vi "pf Init Usb.vi"(8 "error in (no error)":errorcluster, 11 "pDllName":string) -> (0 "error out":errorcluster, 2 "function return":i32, 3 "pDllName out":string)   [LabVIEW 2025, in "Photonfocus_Toolkit.lvlib"]
doc: "PFCONFIG_API int pfInitUsb(char* pDllName);"
uses:
  Photonfocus_Toolkit.lvlib
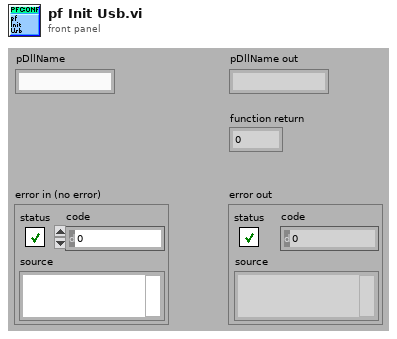
[diagram p1: front panel]
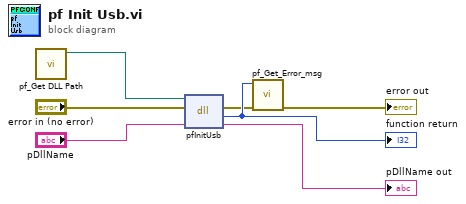
[diagram p0: block diagram]
diagram:
  n1 = call "pf_Get DLL Path.vi"() -> ("DLL path"=w1:path)  [unwired: 1 in, 10 out]
  n2 = dll-call lib="S:/Progetti/Photonfocus/Codice/DEV/PFConfig_lvlib/PFConfig.*" fn="pfInitUsb"(path in=w1, error in="error in (no error)", "pDllName"="pDllName") -> (error out=w3:errorcluster, "return type"=w7:i32, "pDllName"=→"pDllName out":string)  [unwired: 1 in, 1 out]
  "function return" <- w7
  n3 = call "pf_Get_Error_msg.vi"("error in (no error)"=w3, "error code"=w7) -> ("error out"=→"error out":errorcluster)  [unwired: 1 in, 8 out]
